vi "joystick_get_pressed.vi"(6 "Scaler":i8=127, 9 "JoystickDevRef":T3={"Device"=enum."USB 1"}) -> (0 "Buttons Pressed?":bool[](array[boolean]), 1 "Buttons":T1, 2 "Axes":T2, 3 "JoystickDevRef":T3={"Device"=enum."USB 1"}, 4 "POVs":i16[](array[numeric]))   [LabVIEW 2014]
uses:
  <vilib>/Rock Robotics/WPI/Joystick/WPI_JoystickDevRef.ctl
  <vilib>/Rock Robotics/WPI/Joystick/WPI_JoystickDeviceEnum.ctl
  typedefs/joystick_buttons.ctl
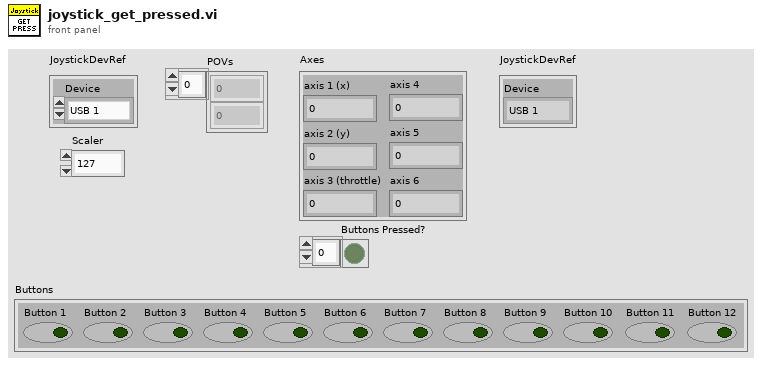
[diagram p1: front panel]
types:
  T1 = typedef "joystick_buttons.ctl" = cluster{"Button 1":bool, "Button 2":bool, "Button 3":bool, "Button 4":bool, "Button 5":bool, "Button 6":bool, "Button 7":bool, "Button 8":bool, "Button 9":bool, "Button 10":bool, "Button 11":bool, "Button 12":bool}
  T2 = cluster{"axis 1 (x)":dbl, "axis 2 (y)":dbl, "axis 3 (throttle)":dbl, "axis 4":dbl, "axis 5":dbl, "axis 6":dbl}
  T3 = typedef "WPI_JoystickDevRef.ctl" = cluster{"Device":T4}
  T4 = typedef "WPI_JoystickDeviceEnum.ctl" = enum16{"USB 0", "USB 1", "USB 2", "USB 3", "USB 4", "USB 5"}
  T5 = cluster{"axis 1 (x)":dbl, "axis 2 (y)":dbl, "axis 3 (z)":dbl, "axis 4 (twist)":dbl, "axis 5 (throttle)":dbl, "axis 6 (num)":dbl}
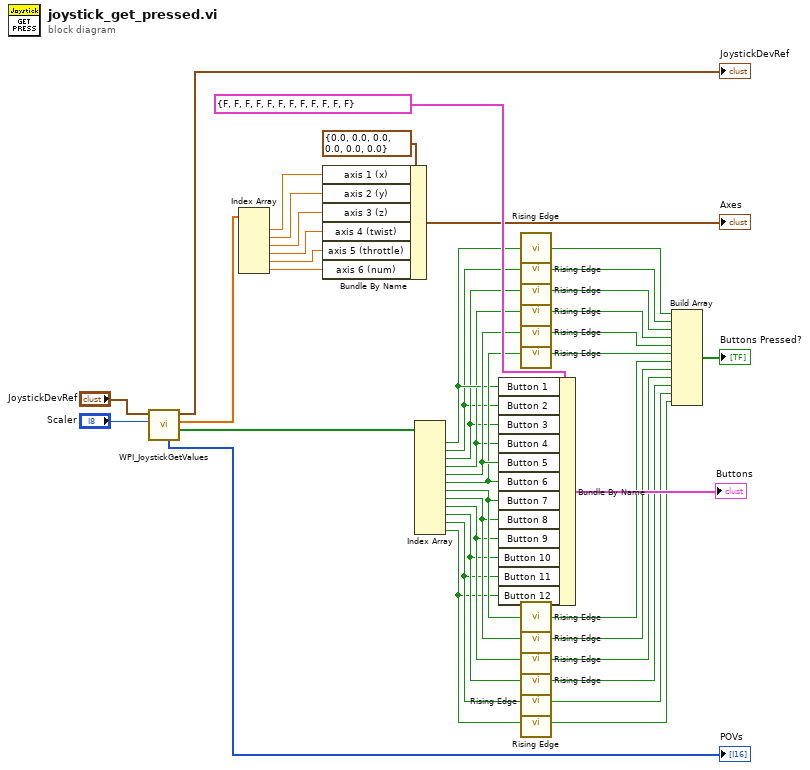
[diagram p0: block diagram]
diagram:
  n1 = call <vilib>:"WPI_JoystickGetValues.vi"("Scaler"="Scaler", "JoystickDevRef"="JoystickDevRef") -> ("Buttons"=w21:bool[], "Axes"=w8:dbl[], "JoystickDevRef"=→"JoystickDevRef":T3, "POVs"=→"POVs":i16[])  [unwired: 5 in, 1 out]
  n2 = Index Array(array=w8) -> (element #1=w7:dbl, element #2=w6:dbl, element #3=w5:dbl, element #4=w4:dbl, element #5=w3:dbl, element #6=w2:dbl)  [unwired: 6 in]
  n3 = Bundle By Name(cluster=T5 {"axis 1 (x)"=0.0, "axis 2 (y)"=0.0, "axis 3 (z)"=0.0, "axis 4 (twist)"=0.0, "axis 5 (throttle)"=0.0, "axis 6 (num)"=0.0} ("Axes"), "axis 1 (x)"=w7, "axis 2 (y)"=w6, "axis 3 (z)"=w5, "axis 4 (twist)"=w4, "axis 5 (throttle)"=w3, "axis 6 (num)"=w2) -> (→"Axes":T5)
  n4 = Index Array(array=w21) -> (element #1=w20:bool, element #2=w17:bool, element #3=w18:bool, element #4=w19:bool, element #5=w25:bool, element #6=w24:bool, element #7=w23:bool, element #8=w16:bool, element #9=w15:bool, element #10=w14:bool, element #11=w13:bool, element #12=w12:bool)  [unwired: 12 in]
  n5 = Bundle By Name(cluster=T1 {"Button 1"=FALSE, "Button 2"=FALSE, "Button 3"=FALSE, "Button 4"=FALSE, "Button 5"=FALSE, "Button 6"=FALSE, "Button 7"=FALSE, "Button 8"=FALSE, "Button 9"=FALSE, "Button 10"=FALSE, "Button 11"=FALSE, "Button 12"=FALSE} ("Buttons"), "Button 1"=w20, "Button 2"=w17, "Button 3"=w18, "Button 4"=w19, "Button 5"=w25, "Button 6"=w24, "Button 7"=w23, "Button 8"=w16, "Button 9"=w15, "Button 10"=w14, "Button 11"=w13, "Button 12"=w12) -> (→"Buttons":T1)
  n6 = call "Rising Edge.vi"("Input"=w20) -> ("Rising Edge"=w37:bool)
  n7 = call "Rising Edge.vi"("Input"=w17) -> ("Rising Edge"=w36:bool)
  n8 = call "Rising Edge.vi"("Input"=w18) -> ("Rising Edge"=w35:bool)
  n9 = call "Rising Edge.vi"("Input"=w19) -> ("Rising Edge"=w34:bool)
  n10 = call "Rising Edge.vi"("Input"=w25) -> ("Rising Edge"=w33:bool)
  n11 = call "Rising Edge.vi"("Input"=w24) -> ("Rising Edge"=w32:bool)
  n12 = call "Rising Edge.vi"("Input"=w23) -> ("Rising Edge"=w31:bool)
  n13 = call "Rising Edge.vi"("Input"=w16) -> ("Rising Edge"=w30:bool)
  n14 = call "Rising Edge.vi"("Input"=w15) -> ("Rising Edge"=w29:bool)
  n15 = call "Rising Edge.vi"("Input"=w14) -> ("Rising Edge"=w28:bool)
  n16 = call "Rising Edge.vi"("Input"=w13) -> ("Rising Edge"=w27:bool)
  n17 = call "Rising Edge.vi"("Input"=w12) -> ("Rising Edge"=w26:bool)
  n18 = Build Array(w37, w36, w35, w34, w33, w32, w31, w30, w29, w28, w27, w26) -> (→"Buttons Pressed?":bool[])
